vi "2DArraySmooth.vi"(1 "Array":dbl[][](array[numeric]), 2 "Smooth Factor":i32) -> (0 "2D Out":dbl[][](array[numeric]))   [LabVIEW 2015]
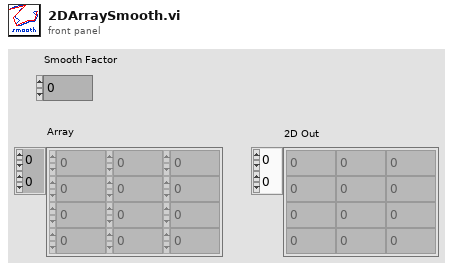
[diagram p1: front panel]
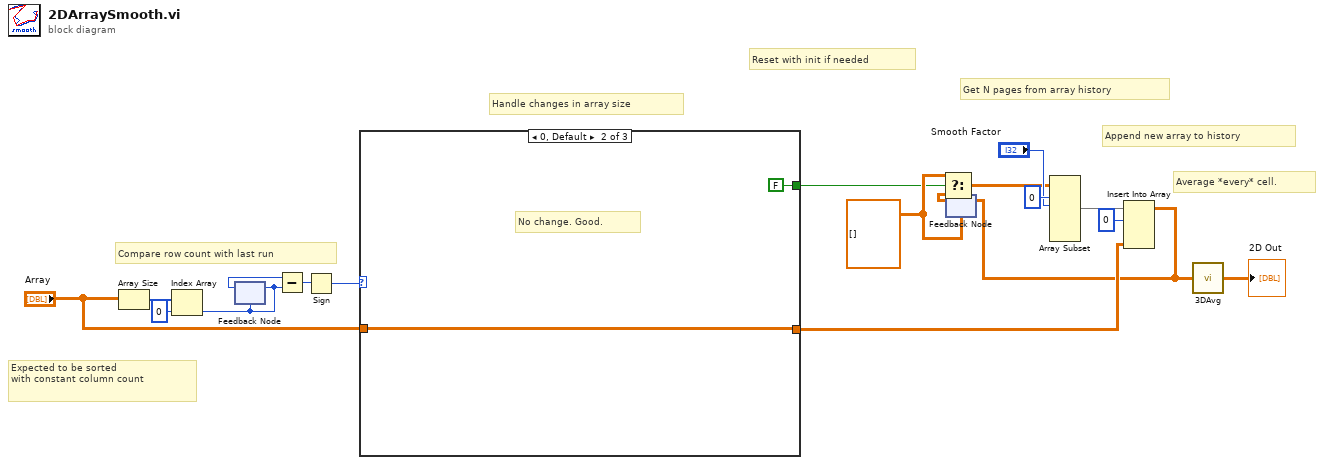
[diagram p0: block diagram]
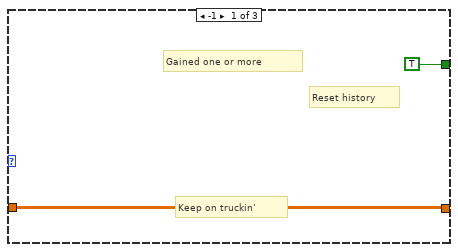
[diagram p2: hidden frame]
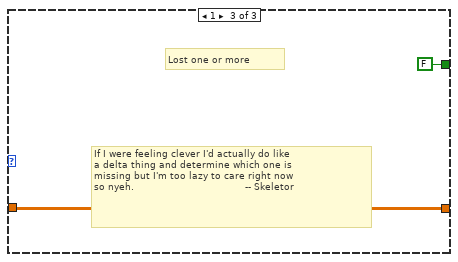
[diagram p3: hidden frame]
diagram:
  w2 = dbl[][][] []
  # "Reset with init if needed"
  # "Handle changes in array size"
  # "Average *every* cell."
  # "Append new array to history"
  # "Get N pages from array history"
  # "Compare row count with last run"
  # "Expected to be sorted\nwith constant column count"
  n1 = Array Size(array="Array") -> (size(s)=w18:i32[])
  n2 = Index Array(array=w18, index=0) -> (element=w8:i32)
  n3 = feedback-in #1(w8) -> ()
  n4 = feedback #1(w8) -> (w7:i32)
  n5 = Subtract(x=w7, y=w8) -> (x-y=w6:i32)
  n6 = Sign(1:w6) -> (0:w5:i32)
  n7 = case shown="0, Default" w5 {
    tunnel: "Array" -> [w19 w22 w23]
    tunnel: [w19 w22 w23] -> w11
    tunnel: [TRUE FALSE FALSE] -> w1
    frame -1 {
      # "Keep on truckin'"
      # "Reset history"
      # "Gained one or more"
    }
    frame 0, Default {
      # "No change. Good."
    }
    frame 1 {
      # "If I were feeling clever I'd actually do like\na delta thing and determine which one is\nmissing but I'm too lazy to care right now\nso nyeh.                                     -- Skeletor"
      # "Lost one or more"
    }
  }
  n8 = feedback #2(w2) -> (w4:dbl[][][])
  n9 = Select(t=w2, s=w1, f=w4) -> (s? t:f=w3:dbl[][][])
  n10 = Array Subset(array=w3, index (dim 0)=0 ("index"), length (dim 0)="Smooth Factor") -> (w12:dbl[][][])  [unwired: 4 in]
  n11 = Insert Into Array(array=w12, index (dim 0)=0 ("index"), new element=w11) -> (w10:dbl[][][])  [unwired: 2 in]
  n12 = feedback-in #2(w10) -> ()
  n13 = call "3DAvg.vi"("3D In"=w10) -> ("2D Out"=→"2D Out":dbl[][])
